vi "Pelco_D_cmd.vi"() -> ()   [LabVIEW 2018]
panel:
  in  "query. query magnification":string="ÿ\u0002\u0000K\u0000\u0000M"
  in  "query.set magnification":string="ÿ\u0002\u0000K\u0000\u0000M"
  in  "query.cam default":string="ÿ\u0002\u0000K\u0000\u0000M"
  in  "query.set position tilt zero":string="ÿ\u0002\u0000M\u0000\u0000O"
  in  "query.set position pan zero":string="ÿ\u0002\u0000K\u0000\u0000M"
  in  "queery.stop cmd":string="ÿ\u0001\u0000\u0000\u0000\u0000\u0001"
  in  "query.pan position":string="ÿ\u0002\u0000Q\u0000\u0000S"
  in  "query.tilt position":string="ÿ\u0002\u0000S\u0000\u0000U"
  in  "query.go to zero pan":string="ÿ\u0001\u0000\u0007\u0000\"\n"
  in  "queery.remote reset":string="ÿ\u0002\u0000\u000f\u0000\u0000\u0011"
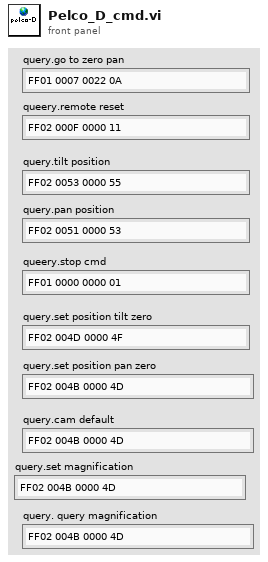
[diagram p1: front panel]
diagram:
